vi "Set Inhibited On.vi"(8 "error in (no error)":errorcluster, 11 "VISA resource name":refnum<visa-resource-name>="COM1") -> (0 "error out":errorcluster, 2 "query output":string, 3 "VISA resource name out":refnum<visa-resource-name>)   [LabVIEW 2017]
panel:
  out "Numeric":i32
  out "read buffer":string
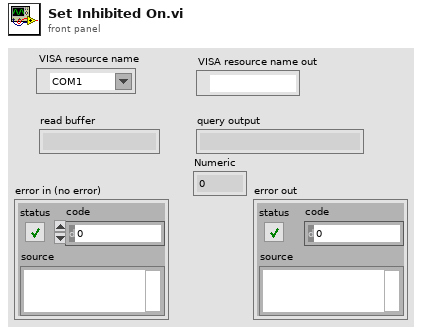
[diagram p1: front panel]
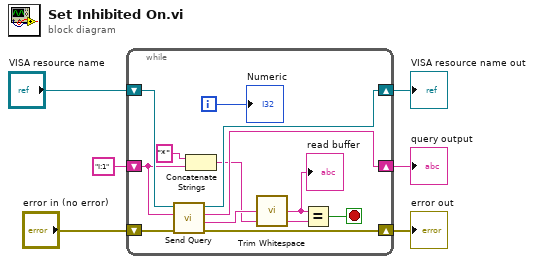
[diagram p0: block diagram]
diagram:
  n1 = while {
    shift-right: [w16] -> w3
    shift-left: "VISA resource name" -> [w18]
    shift-right: [w14] -> w1
    shift-left: "I:1" ("query string") -> [w12]
    shift-right: [w15] -> w2
    shift-left: "error in (no error)" -> [w17]
    i -> [w7]
    stop <- w8 stop-if-true
    n2 = call "Send Query.vi"("error in (no error)"=w17, "query string"=w12, "VISA resource name"=w18) -> ("error out"=w15:errorcluster, "read buffer"=w13:string, "query output"=w14:string, "VISA resource name out"=w16:refnum<visa-resource-name>)  [unwired: 5 in]
    n3 = Concatenate Strings("*" ("string"), w12) -> (w9:string)
    n4 = call <vilib>:"Trim Whitespace.vi"("string"=w13) -> ("trimmed string"=w10:string)  [unwired: 1 in]
    "read buffer" <- w10
    n5 = Equal?(x=w10, y=w9) -> (x = y?=w8:bool)
    "Numeric" <- w7
  }
  "error out" <- w2
  "VISA resource name out" <- w3
  "query output" <- w1
